vi "main.vi"(2 "depth":dbl=130.0, 3 "rotation":dbl[](array[numeric]) step=0.1) -> ()   [LabVIEW 2018]
uses:
  <vilib>/Platform/TimedLoop/XDataNode/timing_clust.ctl
  <vilib>/Platform/TimedLoop/XDataNode/nitl_modes.ctl
  <vilib>/Platform/TimedLoop/XDataNode/wakeup.ctl
  <vilib>/myRIO/Common/Instrument Driver Framework/myRIO v1.0/Encoder/typedefs/Encoder Signal Mode.ctl
  <vilib>/myRIO/Instrument Drivers/Onboard IO/Encoder/typedefs/Encoder Reference.ctl
  <vilib>/myRIO/Common/Instrument Driver Framework/Utilities/typedefs/myRIO Generic Hardware Reference.ctl
  <vilib>/myRIO/Common/Instrument Driver Framework/Utilities/typedefs/Hardware Version Enum.ctl
  <vilib>/myRIO/Common/Instrument Driver Framework/Utilities/typedefs/myRIO v1.0 Reference.ctl
  <vilib>/myRIO/Common/Instrument Driver Framework/Utilities/typedefs/Generic FPGA Reference.ctl
  <vilib>/myRIO/Common/Instrument Driver Framework/myRIO v1.0/Encoder/typedefs/Encoder Channels Enum.ctl
  <vilib>/myRIO/Common/Instrument Driver Framework/myRIO v1.0/Encoder/typedefs/Encoder Configuration v1.0.ctl
  <vilib>/userdefined/High Color/nirio_resource_hc.ctl
  <vilib>/myRIO/Common/Instrument Driver Framework/Utilities/vis/Is FPGA Ref Available.vi
  <vilib>/myRIO/Common/Instrument Driver Framework/myRIO v1.0/Encoder/vis/myRIO v1.1 Open Encoder.vi
  <vilib>/myRIO/Instrument Drivers/Onboard IO/Encoder/vis/Read.vi
  <vilib>/myRIO/Common/Instrument Driver Framework/Utilities/vis/Validate Channels.vi
  <vilib>/myRIO/Common/Instrument Driver Framework/myRIO v1.0/Encoder/vis/myRIO v1.0 Reserve Encoder.vi
  <vilib>/myRIO/Common/Instrument Driver Framework/myRIO v1.0/Encoder/vis/myRIO v1.0 Build MUX Configuration Encoder.vi
  <vilib>/myRIO/Common/Instrument Driver Framework/myRIO v1.0/Resource Manager/vis/myRIO v1.0 Reserve Channel List.vi
  <vilib>/myRIO/Common/Instrument Driver Framework/myRIO v1.0/Resource Manager/vis/myRIO v1.0 Create Configuration List.vi
  <vilib>/myRIO/Common/Instrument Driver Framework/myRIO v1.0/Resource Manager/vis/myRIO v1.0 Reserve Channel.vi
  <vilib>/myRIO/Common/Instrument Driver Framework/myRIO v1.0/Resource Manager/vis/myRIO v1.0 Unreserve Channel.vi
  <vilib>/myRIO/Common/Instrument Driver Framework/myRIO v1.0/Resource Manager/vis/myRIO v1.0 Build Mutex Name.vi
  <vilib>/FPGAPlugInAG/myRIO-1900/niLvFpga_Open_myRIO-1900.vi
  <vilib>/rvi/interface/common/dynamic/niFpgaDynamicAddResources.vi
  <vilib>/Utility/VariantDataType/GetNumericInfo.vi
  <vilib>/Utility/error.llb/Error Cluster From Error Code.vi
  <vilib>/myRIO/Common/Instrument Driver Framework/myRIO v1.0/myRIO v1.1 Open.vi
  <vilib>/myRIO/Common/Instrument Driver Framework/Utilities/vis/IO Manager.vi
  <vilib>/myRIO/Common/Instrument Driver Framework/Utilities/vis/Configuration Manager.vi
  <vilib>/myRIO/Common/Instrument Driver Framework/myRIO v1.0/Resource Manager/vis/myRIO v1.0 Configure IO.vi
  <vilib>/myRIO/Common/Instrument Driver Framework/myRIO v1.0/myRIO v1.0 Close.vi
  <vilib>/myRIO/Common/Instrument Driver Framework/myRIO v1.0/Encoder/vis/myRIO v1.0 Configure Encoder.vi
  <vilib>/myRIO/Common/Instrument Driver Framework/myRIO v1.0/Encoder/vis/myRIO v1.0 Read Encoder.vi
  <vilib>/rvi/errors/niLvFpgaAdjustHostInterfaceError.vi
  <vilib>/rvi/interface/nirviOpenFPGA/nirviOpenFPGA.xnode
  FPGA Bitfiles/STW_FPGATarget_motercontrol_I8R9CeC8UVc.lvbitx
  motercontrol.vi
  <vilib>/Platform/TimedLoop/XDataNode/XDataNode.xnode
  <vilib>/myRIO/Express VI/Onboard IO/Encoder/Encoder Express VI.xnode
  <vilib>/myRIO/Instrument Drivers/Onboard IO/Encoder/vis/myRIO Encoder Open.xnode
  <vilib>/rvi/interface/nirviReadWriteControl/nirviReadWriteControl.xnode
  <vilib>/Platform/TimedLoop/XDataNode/XDNodeRunTimeDep.lvlib
  NiFpgaLv.dll
  <vilib>/rvi/interface/Simulation/niFpgaSimulationCallBeginRW.vi
  <vilib>/myRIO/Instrument Drivers/Onboard IO/Encoder/Encoder.lvlib
panel:
  out "Counter Direction":enum16{"Counting Up", "Counting Down"}(ring)
  out "encoder count":i32
  out "enable  rotation correction":bool
  in  "rotation control":dbl[](array[slide]) min=-0.5 max=0.5 step=0.05 scale=-0.5..0.5
  out "position":dbl[](array[numeric])
  in  "depth  operation":cluster{"up":bool, "down":bool}
  in  "control source":bool
  in  "listening port":u16=60006
  out "client IP address":string
  out "client port":u16
  out "Ref Array":dbl[](array[numeric])=[0.0, 0.0, 0.0, 0.0, 6000.0]
  in  "Stop Program":bool
  in  "yaw_max":dbl=3.1415
  in  "roll_max":dbl=0.5236
  in  "pitch_min":dbl=-0.6981
  in  "pitch_max":dbl=0.3
  out "Servo Duty Cycle":dbl(slide)=0.07533838383838383 scale=0.07175..0.079
  in  "Servo Period (Ticks)":u32=800000
  out "length":dbl[](array[numeric])
  out "long length_max":dbl
  in  "long length_min":dbl=97.0
  out "result":dbl[][](array[numeric])
  in  "range":dbl=30.0
  out "out len 3":dbl
  out "out len 2":dbl
  out "out len 1":dbl
  out "length_max":dbl=112.0
  in  "length_min":dbl=82.0
  out "Duty Cycle 3":dbl(slide) scale=0.0..1.0
  out "Duty Cycle 2":dbl(slide) scale=0.0..1.0
  in  "Period (Ticks)":u32=100
  out "Duty Cycle":dbl(slide) scale=0.0..1.0
  # "(in rad/s)\nalpha\n\nbeta\n\ngamma"
  # "null"
  # "alpha"
  # "beta"
  # "yaw"
  # "length"
  # "extend/retract"
  # "(rad)"
  # "local / remote"
  # "(amplitude)"
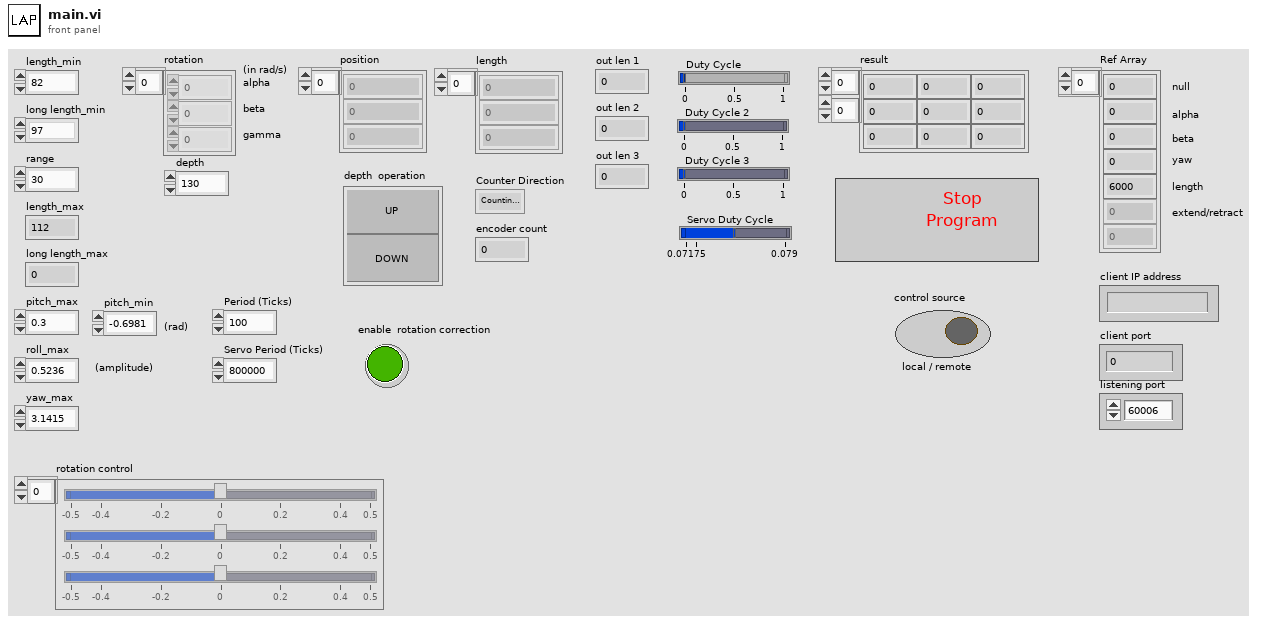
[diagram p1: front panel]
types:
  T1 = typedef "XDNodeRunTimeDep.lvlib/timing_clust.ctl" = cluster{"Expected End [f-1]":u64, "Actual End [f-1]":u64, "Finished Late? [f-1]":bool, "Expected End [i-1]":u64, "Actual End [i-1]":u64, "Finished Late? [i-1]":bool, "Expected Start [i]":u64, "Actual Start [i]":u64, "Expected Start [f]":u64, "Actual Start [f]":u64, "Source Name":string, "Structure Name":string, "Period":i64, "Deadline":i64, "Offset":i64, "Start":i64, "Priority":i32, "Timeout":i32, "Mode":T2, "Wakeup Reason":T3, "Error":errorcluster, "Source Type":string, "Secondary Source Type":string, "Global End Time":u64, "Global Start Time":u64, "Frame Duration":u64, "Iteration Duration":u64, "Assigned CPU":i32, "I/O Scan Engine Mode":u32}
  T2 = typedef "XDNodeRunTimeDep.lvlib/nitl_modes.ctl" = enum32{"No Change", "Process missed periods, maintain original phase", "Discard missed periods, maintain original phase", "Process missed periods, ignore original phase", "Discard missed periods, ignore original phase"}
  T3 = typedef "XDNodeRunTimeDep.lvlib/wakeup.ctl" = enum32{"Normal", "Aborted", "Asynchronous wakeup", "Timing source error", "Timed loop error", "Timeout"}
  T4 = typedef "Encoder.lvlib/Encoder Reference.ctl" = cluster{"myRIO Reference":T5, "Encoder Channels Enum":T9}
  T5 = typedef "myRIO Generic Hardware Reference.ctl" = cluster{"myRIO Model":T6, "myRIO Hardware Reference":T7}
  T6 = typedef "Hardware Version Enum.ctl" = enum16{"Unknown", "myRIO-1900", "myRIO-1950", "roboRIO", "NI ELVIS RIO CM", "ELVIS III"}
  T7 = typedef "myRIO v1.0 Reference.ctl" = cluster{"Generic FPGA Reference":T8, "Allow multiple opens":bool}
  T8 = typedef "Generic FPGA Reference.ctl" = refnum<k20>
  T9 = typedef "Encoder Channels Enum.ctl" = enum16{"Not Connected", "C/ENC0", "C/ENC1", "A/ENC", "A/ENC0", "A/ENC1", "A/ENC2", "A/ENC3", "A/ENC4", "A/ENC5", "A/ENC6", "A/ENC7", "A/ENC8", "A/ENC9", "B/ENC", "B/ENC0", "B/ENC1", "B/ENC2", "B/ENC3", "B/ENC4", "B/ENC5", "B/ENC6", "B/ENC7", "B/ENC8", "B/ENC9", "DIO/ENC0", "DIO/ENC1", "DIO/ENC2", "DIO/ENC3", "DIO/ENC4"}
  T10 = typedef "Encoder Signal Mode.ctl" = enum16{"Quadrature phase signal", "Step and direction signal"}
  T11 = typedef "nirio_resource_hc.ctl" = tag
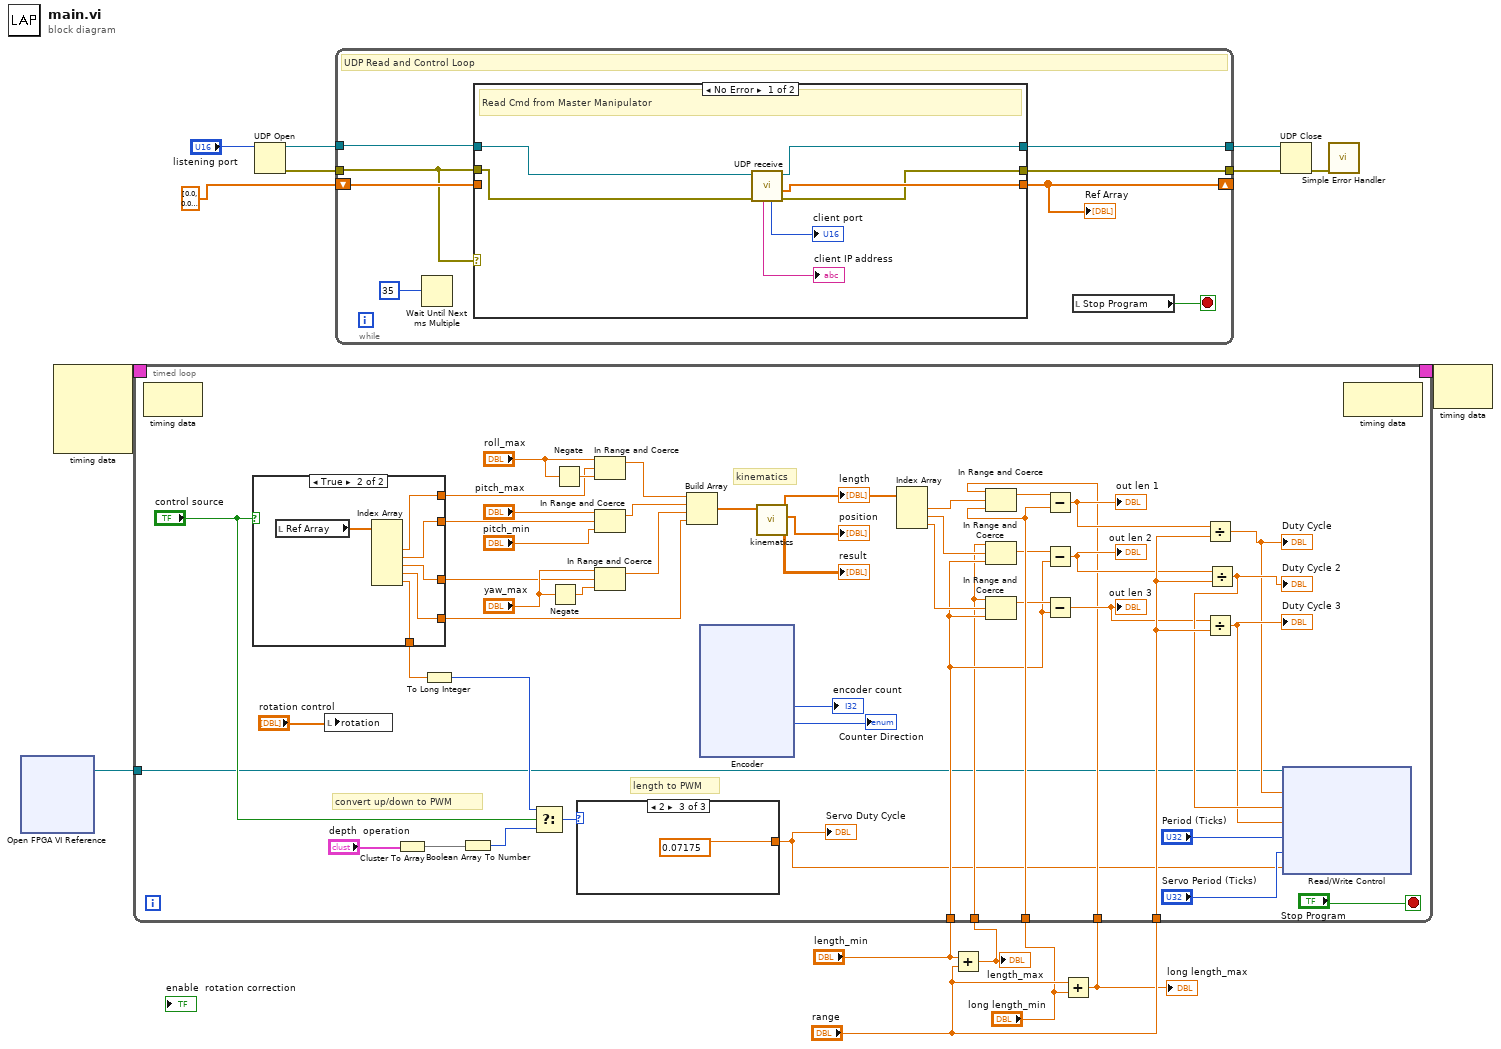
[diagram p0: block diagram]
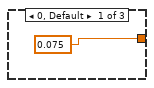
[diagram p3: hidden frame]
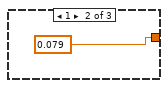
[diagram p4: hidden frame]
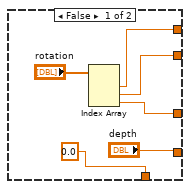
[diagram p5: hidden frame]
diagram:
  n1 = xnode "Open FPGA VI Reference"() -> ("FPGA VI Reference Out"=w13:refnum<k20>)  [unwired: 2 in, 1 out]
  n2 = node-c288() -> (w15:T1)  [unwired: 4 in]
  n3 = UDP Open(11:"listening port") -> (port=w4:refnum<k16>, 0:w3:errorcluster)  [unwired: 4 in, 1 out]
  n4 = while {
    tunnel: w4 -> [w22]
    tunnel: w3 -> [w16]
    tunnel: [w20] -> w7
    tunnel: [w21] -> w6
    shift-right: [w19] -> _
    shift-left: dbl[] [0.0, 0.0, 0.0, 0.0, 0.0] -> [w18]
    stop <- w23 stop-if-true
    # "UDP Read and Control Loop"
    n5 = Wait Until Next ms Multiple(millisecond multiple=u32 35) -> ()  [unwired: 1 out]
    n6 = case shown="No Error" w16 {
      tunnel: w22 -> [w28 w33]
      tunnel: w16 -> [w26 w32]
      tunnel: [w30 w31] -> w19
      tunnel: [w29 w33] -> w21
      tunnel: [w27 w32] -> w20
      tunnel: w18 -> [_ w31]
      frame No Error {
        # "Read Cmd from Master Manipulator"
        n7 = call "UDP receive.vi"("error in"=w26, "UDP connection ID"=w28) -> ("error out"=w27:errorcluster, "Array01"=w30:dbl[], "UDP connection ID out"=w29:refnum<k16>, "client port"=→"client port":u16, "client IP address"=→"client IP address":string)  [unwired: 4 in, 1 out]
      }
      frame Error {
        # "Lost Connection, Keep the Last Cmd as Ref"
      }
    }
    "Ref Array" <- w19
    n8 = local read "Stop Program"() -> (w23:bool)
  }
  n9 = Add(x="length_min", y="range") -> (x+y=w9:dbl)
  "length_max" <- w9
  n10 = Add(x="range", y="long length_min") -> (x+y=w8:dbl)
  "long length_max" <- w8
  n11 = timed-loop "Timed Loop" {
    timing: w15 -> [_]
    timing-out: [_] -> w14
    tunnel: w13 -> [w34]
    tunnel: "length_min" -> [w69]
    tunnel: "range" -> [w81]
    tunnel: "long length_min" -> [w74]
    tunnel: w9 -> [w65]
    tunnel: w8 -> [w64]
    stop <- "Stop Program" stop-if-true
    # "kinematics"
    # "convert up/down to PWM"
    # "length to PWM"
    n12 = node-c288() -> ()  [unwired: 1 in, 1 out]
    n13 = case shown="True" "control source" {
      tunnel: [w136 w142] -> w56
      tunnel: [w135 w141] -> w55
      tunnel: [w134 w140] -> w54
      tunnel: ["depth" w139] -> w47
      tunnel: [0.0 w138] -> w39
      frame False {
        n14 = Index Array(array="rotation") -> (element #1=w136:dbl, element #2=w135:dbl, element #3=w134:dbl)  [unwired: 3 in]
      }
      frame True {
        n15 = local read "Ref Array"() -> (w143:dbl[])
        n16 = Index Array(array=w143) -> (element #2=w142:dbl, element #3=w141:dbl, element #4=w140:dbl, element #5=w139:dbl, element #6=w138:dbl)  [unwired: 6 in, 1 out]
      }
    }
    n17 = local write "rotation"("rotation control") -> ()
    n18 = Cluster To Array(cluster="depth  operation") -> (array=w52:bool[])
    n19 = To Long Integer(number=w39) -> (32bit integer=w38:i32)
    n20 = Boolean Array To Number(Boolean array=w52) -> (number=w41:u32)
    n21 = Select(t=w38, s="control source", f=w41) -> (s? t:f=w40:u32)
    n22 = Negate(x="yaw_max") -> (-x=w76:dbl)
    n23 = Negate(x="roll_max") -> (-x=w58:dbl)
    n24 = case shown="2" w40 {
      tunnel: [0.075 0.079 0.07175] -> w51
      frame 0, Default {
      }
      frame 1 {
      }
      frame 2 {
      }
    }
    "Servo Duty Cycle" <- w51
    n25 = In Range and Coerce(upper limit="roll_max", x=w56, lower limit=w58) -> (coerced(x)=w50:dbl)  [unwired: 1 out]
    n26 = In Range and Coerce(upper limit="pitch_max", x=w55, lower limit="pitch_min") -> (coerced(x)=w49:dbl)  [unwired: 1 out]
    n27 = In Range and Coerce(upper limit="yaw_max", x=w54, lower limit=w76) -> (coerced(x)=w48:dbl)  [unwired: 1 out]
    n28 = Build Array(w50, w49, w48, w47) -> (w46:dbl[])
    n29 = xnode "Encoder"() -> ("Counter Value"=→"encoder count":i32, "Counter Direction"=→"Counter Direction":enum16{"Counting Up", "Counting Down"})  [unwired: 2 in, 2 out]
    n30 = call "kinematics.vi"("input"=w46) -> ("result"=→"result":dbl[][], "position"=→"position":dbl[], "length"=w45:dbl[])  [unwired: 8 in]
    "length" <- w45
    n31 = Index Array(array=w45) -> (element #1=w63:dbl, element #2=w70:dbl, element #3=w71:dbl)  [unwired: 3 in]
    n32 = In Range and Coerce(upper limit=w64, x=w63, lower limit=w74) -> (coerced(x)=w62:dbl)  [unwired: 1 out]
    n33 = In Range and Coerce(upper limit=w65, x=w70, lower limit=w69) -> (coerced(x)=w72:dbl)  [unwired: 1 out]
    n34 = In Range and Coerce(upper limit=w65, x=w71, lower limit=w69) -> (coerced(x)=w73:dbl)  [unwired: 1 out]
    n35 = Subtract(x=w62, y=w74) -> (x-y=w68:dbl)
    "out len 1" <- w68
    n36 = Subtract(x=w72, y=w69) -> (x-y=w67:dbl)
    "out len 2" <- w67
    n37 = Subtract(x=w73, y=w69) -> (x-y=w66:dbl)
    "out len 3" <- w66
    n38 = Divide(x=w68, y=w81) -> (x/y=w77:dbl)
    "Duty Cycle" <- w77
    n39 = Divide(x=w66, y=w81) -> (x/y=w79:dbl)
    "Duty Cycle 3" <- w79
    n40 = Divide(x=w67, y=w81) -> (x/y=w80:dbl)
    "Duty Cycle 2" <- w80
    n41 = xnode "Read/Write Control"("FPGA VI Reference In"=w34, "Duty Cycle"=w77, "Duty Cycle 2"=w80, "Duty Cycle 3"=w79, "Period (Ticks)"="Period (Ticks)", "Servo Period (Ticks)"="Servo Period (Ticks)", "Servo Duty Cycle"=w51) -> ()  [unwired: 1 in, 2 out]
    n42 = node-c288() -> ()  [unwired: 1 in, 1 out]
  }
  n43 = UDP Close(connection ID=w6, 8:w7) -> (error out=w1:errorcluster)  [unwired: 1 out]
  n44 = call <vilib>:"Simple Error Handler.vi"("error in (no error)"=w1) -> ()  [unwired: 4 in, 5 out]
  n45 = node-c288(w14) -> ()  [unwired: 1 out]
